vi "LuaVIEW Cleanup Registry_srv.vi"(7 "certificate":string) -> (15 "error out":errorcluster)   [LabVIEW 2012]
uses:
  clientsrv/typedefs/t_ClientSrv Access Levels.ctl
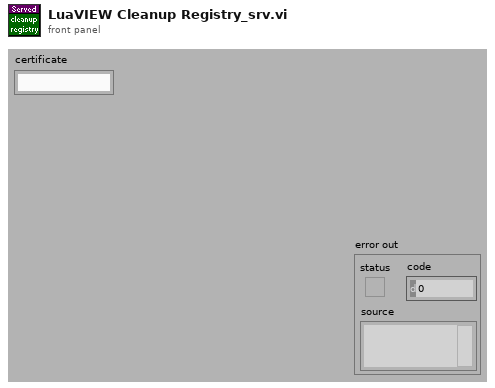
[diagram p1: front panel]
types:
  T1 = typedef "t_ClientSrv Access Levels.ctl" = enum16{"observer", "operator", "local"}
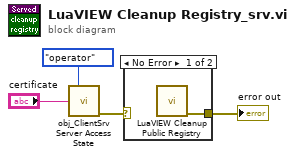
[diagram p0: block diagram]
diagram:
  n1 = call "obj_ClientSrv Server Access State.vi"("access level"=t_ClientSrv_Access_Levels."operator", "certificate in"="certificate") -> ("error out"=w2:errorcluster)  [unwired: 11 in, 2 out]
  n2 = case shown="No Error" w2 {
    selector: w2 -> [_ w6]
    tunnel: [w5 w6] -> w1
    frame No Error {
      n3 = call "LuaVIEW Cleanup Public Registry.vi"() -> ("error out"=w5:errorcluster)  [unwired: 15 in]
    }
    frame Error {
    }
  }
  "error out" <- w1
